vi "ExMoveSpectro.vi"() -> ()   [LabVIEW 2010]
panel:
  out "Current Wavelength":string
  in  "Increment Wavelength":dbl=50.0 format="%.2f"
  in  "End Wavelength":dbl=700.0 format="%.2f"
  in  "Start Wavelength":dbl format="%.2f"
  in  "Grating Speed":dbl=2000.0 min=1.0 step=1.0 format="%.2f"
  in  "Grating number":i16=1 min=1 max=100 step=1
  out "error out":errorcluster
  in  "error in (no error)":errorcluster
  # "ExMoveSpectro.vi\n(Normal Spectrograph via USB/COM port)\nThis VI is a simple example of how to setup and move a spectrograph in increments over a wavelength range."
  # "NOTES:\nA properly configured spectometer .ini must be present in the LabVIEW folder for spectrograph operation.\n\nConsult the Toolkit documentation for more information on how to configure this file."
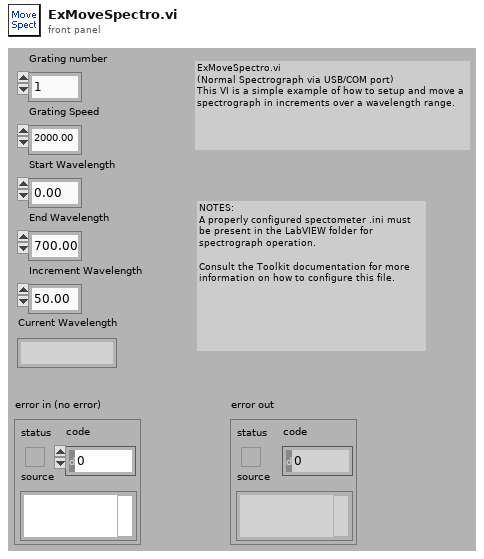
[diagram p1: front panel]
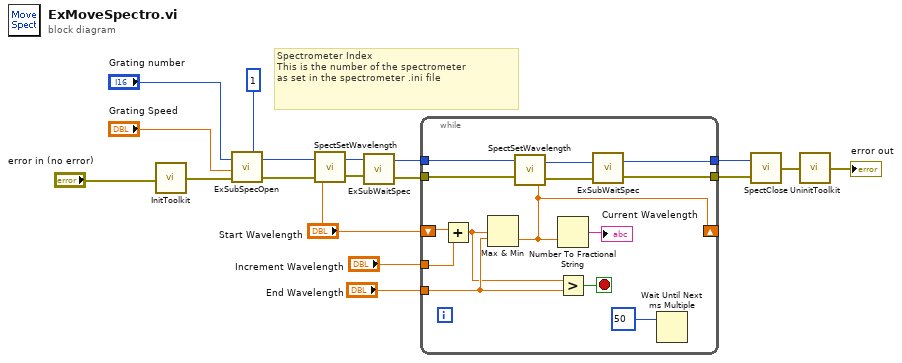
[diagram p0: block diagram]
diagram:
  # "Spectrometer Index\nThis is the number of the spectrometer\nas set in the spectrometer .ini file"
  n1 = call <userlib>:"InitToolkit.vi"("error in"="error in (no error)") -> ("error out"=w1:errorcluster)
  n2 = call "ExSubSpecOpen.vi"("error in (no error)"=w1, "Grating speed"="Grating Speed", "Grating number"="Grating number", "Camera Handles"=1) -> ("error out"=w8:errorcluster, "Spectrometer Handle"=w12:u32)  [unwired: 1 out]
  n3 = call <userlib>:"SpectSetWavelength.vi"("error in"=w8, "Wavelength"="Start Wavelength", "Spectrometer Handle"=w12) -> ("error out"=w16:errorcluster, "Spectrumeter Handle"=w15:u32)
  n4 = call "ExSubWaitSpec.vi"("error in (no error)"=w16, "Spectrometer Handle"=w15) -> ("error out"=w6:errorcluster, "Spectrometer handle"=w14:u32)
  n5 = while {
    tunnel: w14 -> [w23]
    tunnel: "Increment Wavelength" -> [w30]
    tunnel: "End Wavelength" -> [w22]
    shift-right: [w20] -> _
    shift-left: "Start Wavelength" -> [w31]
    tunnel: [w27] -> w9
    tunnel: [w24] -> w7
    tunnel: w6 -> [w26]
    stop <- w21 stop-if-true
    n6 = Add(x=w31, y=w30) -> (x+y=w19:dbl)
    n7 = Max & Min(x=w19, y=w22) -> (min(x,y)=w20:dbl)  [unwired: 1 out]
    n8 = call <userlib>:"SpectSetWavelength.vi"("error in"=w26, "Wavelength"=w20, "Spectrometer Handle"=w23) -> ("error out"=w25:errorcluster, "Spectrumeter Handle"=w28:u32)
    n9 = Number To Fractional String(number=w20) -> (F-format string=→"Current Wavelength":string)  [unwired: 3 in]
    n10 = Greater?(x=w19, y=w22) -> (0:w21:bool)
    n11 = call "ExSubWaitSpec.vi"("error in (no error)"=w25, "Spectrometer Handle"=w28) -> ("error out"=w24:errorcluster, "Spectrometer handle"=w27:u32)
    n12 = Wait Until Next ms Multiple(millisecond multiple=50) -> ()  [unwired: 1 out]
  }
  n13 = call <userlib>:"SpectClose.vi"("error in"=w7, "Spectrometer Handle"=w9) -> ("error out"=w3:errorcluster)
  n14 = call <userlib>:"UninitToolkit.vi"("error in"=w3) -> ("error out"=→"error out":errorcluster)
